vi "Read Index.vi"(8 "error in (no error)":errorcluster, 11 "Socket in":refnum<class "Execution.lvclass">) -> (0 "error out":errorcluster, 2 "Index":u8, 3 "Socket out":refnum<class "Execution.lvclass">)   [LabVIEW 2015, in "Execution.lvclass"]
uses:
  Execution.lvclass
  Execution.lvclass/Execution.ctl
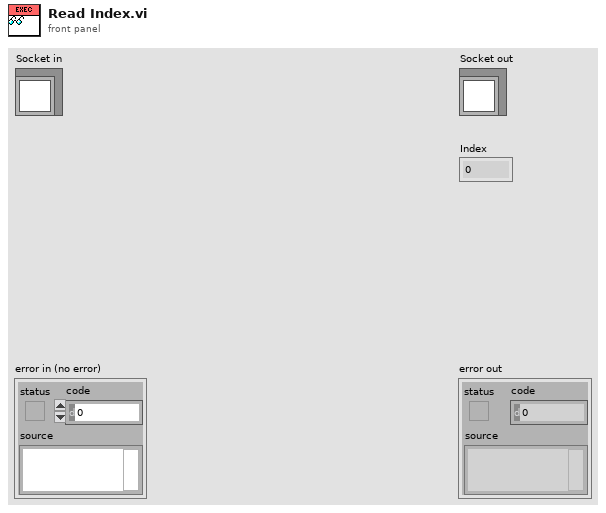
[diagram p1: front panel]
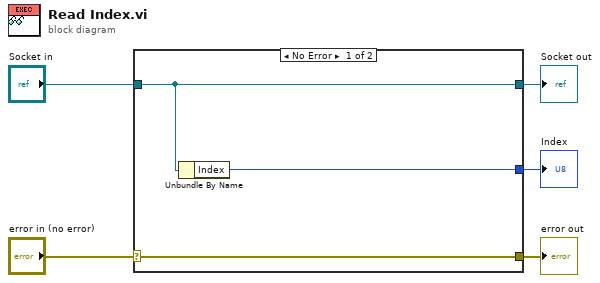
[diagram p0: block diagram]
diagram:
  n1 = case shown="No Error" "error in (no error)" {
    selector: "error in (no error)" -> [w8 w9]
    tunnel: [w8 w9] -> w4
    tunnel: [w7 w10] -> w2
    tunnel: "Socket in" -> [w7 w10]
    tunnel: [w6 _] -> w1
    frame No Error {
      n2 = Unbundle By Name(w7) -> ("Index"=w6:u8)
    }
    frame Error {
    }
  }
  "error out" <- w4
  "Socket out" <- w2
  "Index" <- w1
